vi "new FGGA TCP Packet_v3.3.vi"(0 "ID":string, 5 "Version":string, 7 "TCP Packet In":string, 9 "utc_time":u32, 12 "Data Array":string[](array[string])) -> (8 "TCP Binary Packet":string)   [LabVIEW 2014]
panel:
  out "array":string[](array[string])
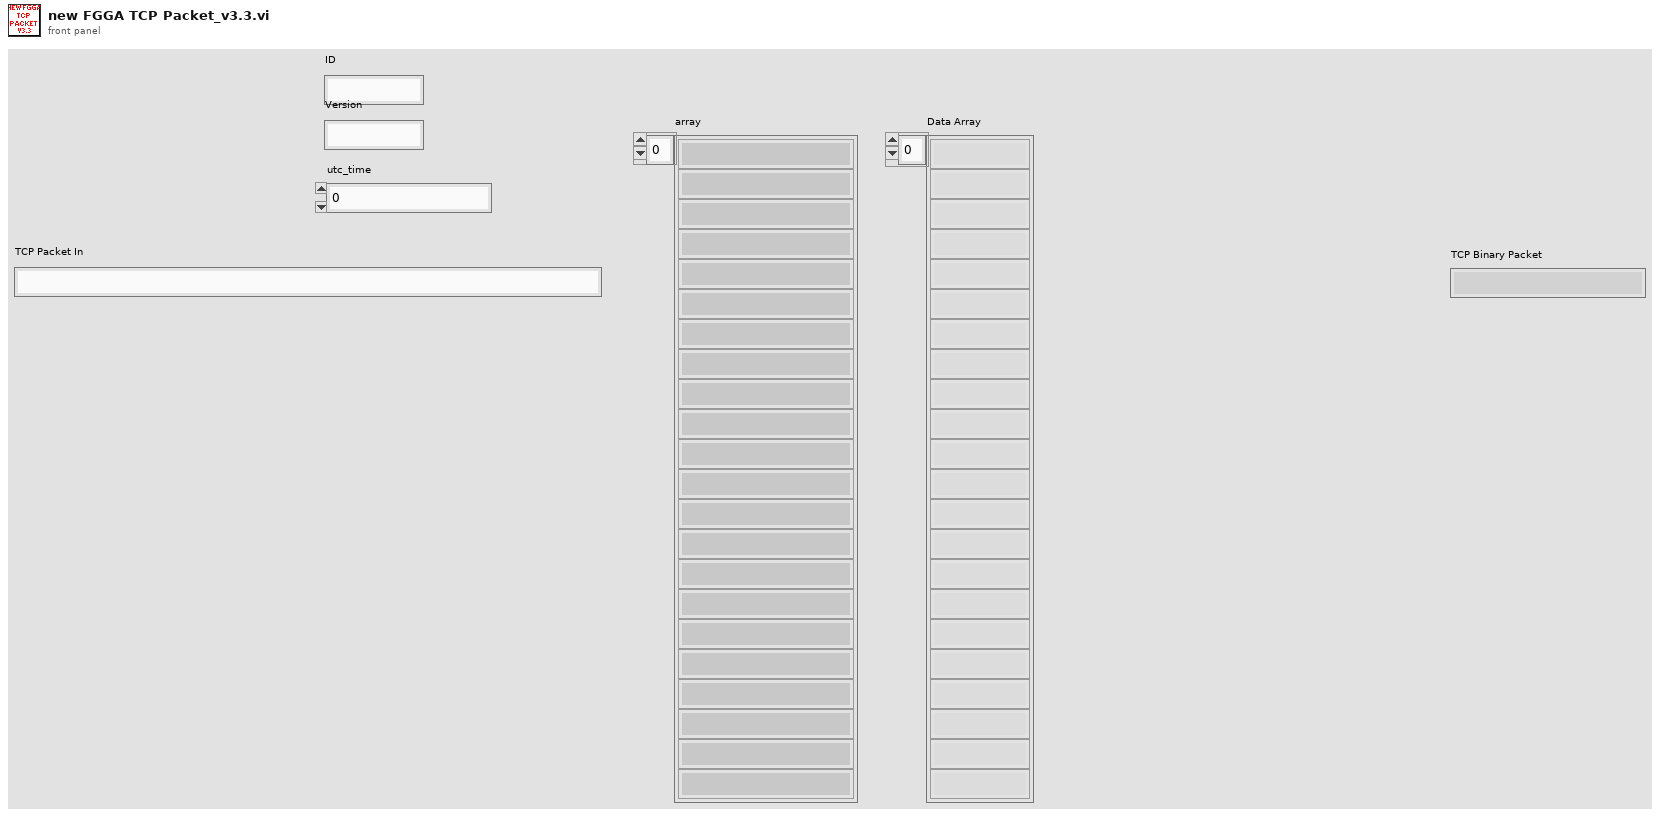
[diagram p1: front panel]
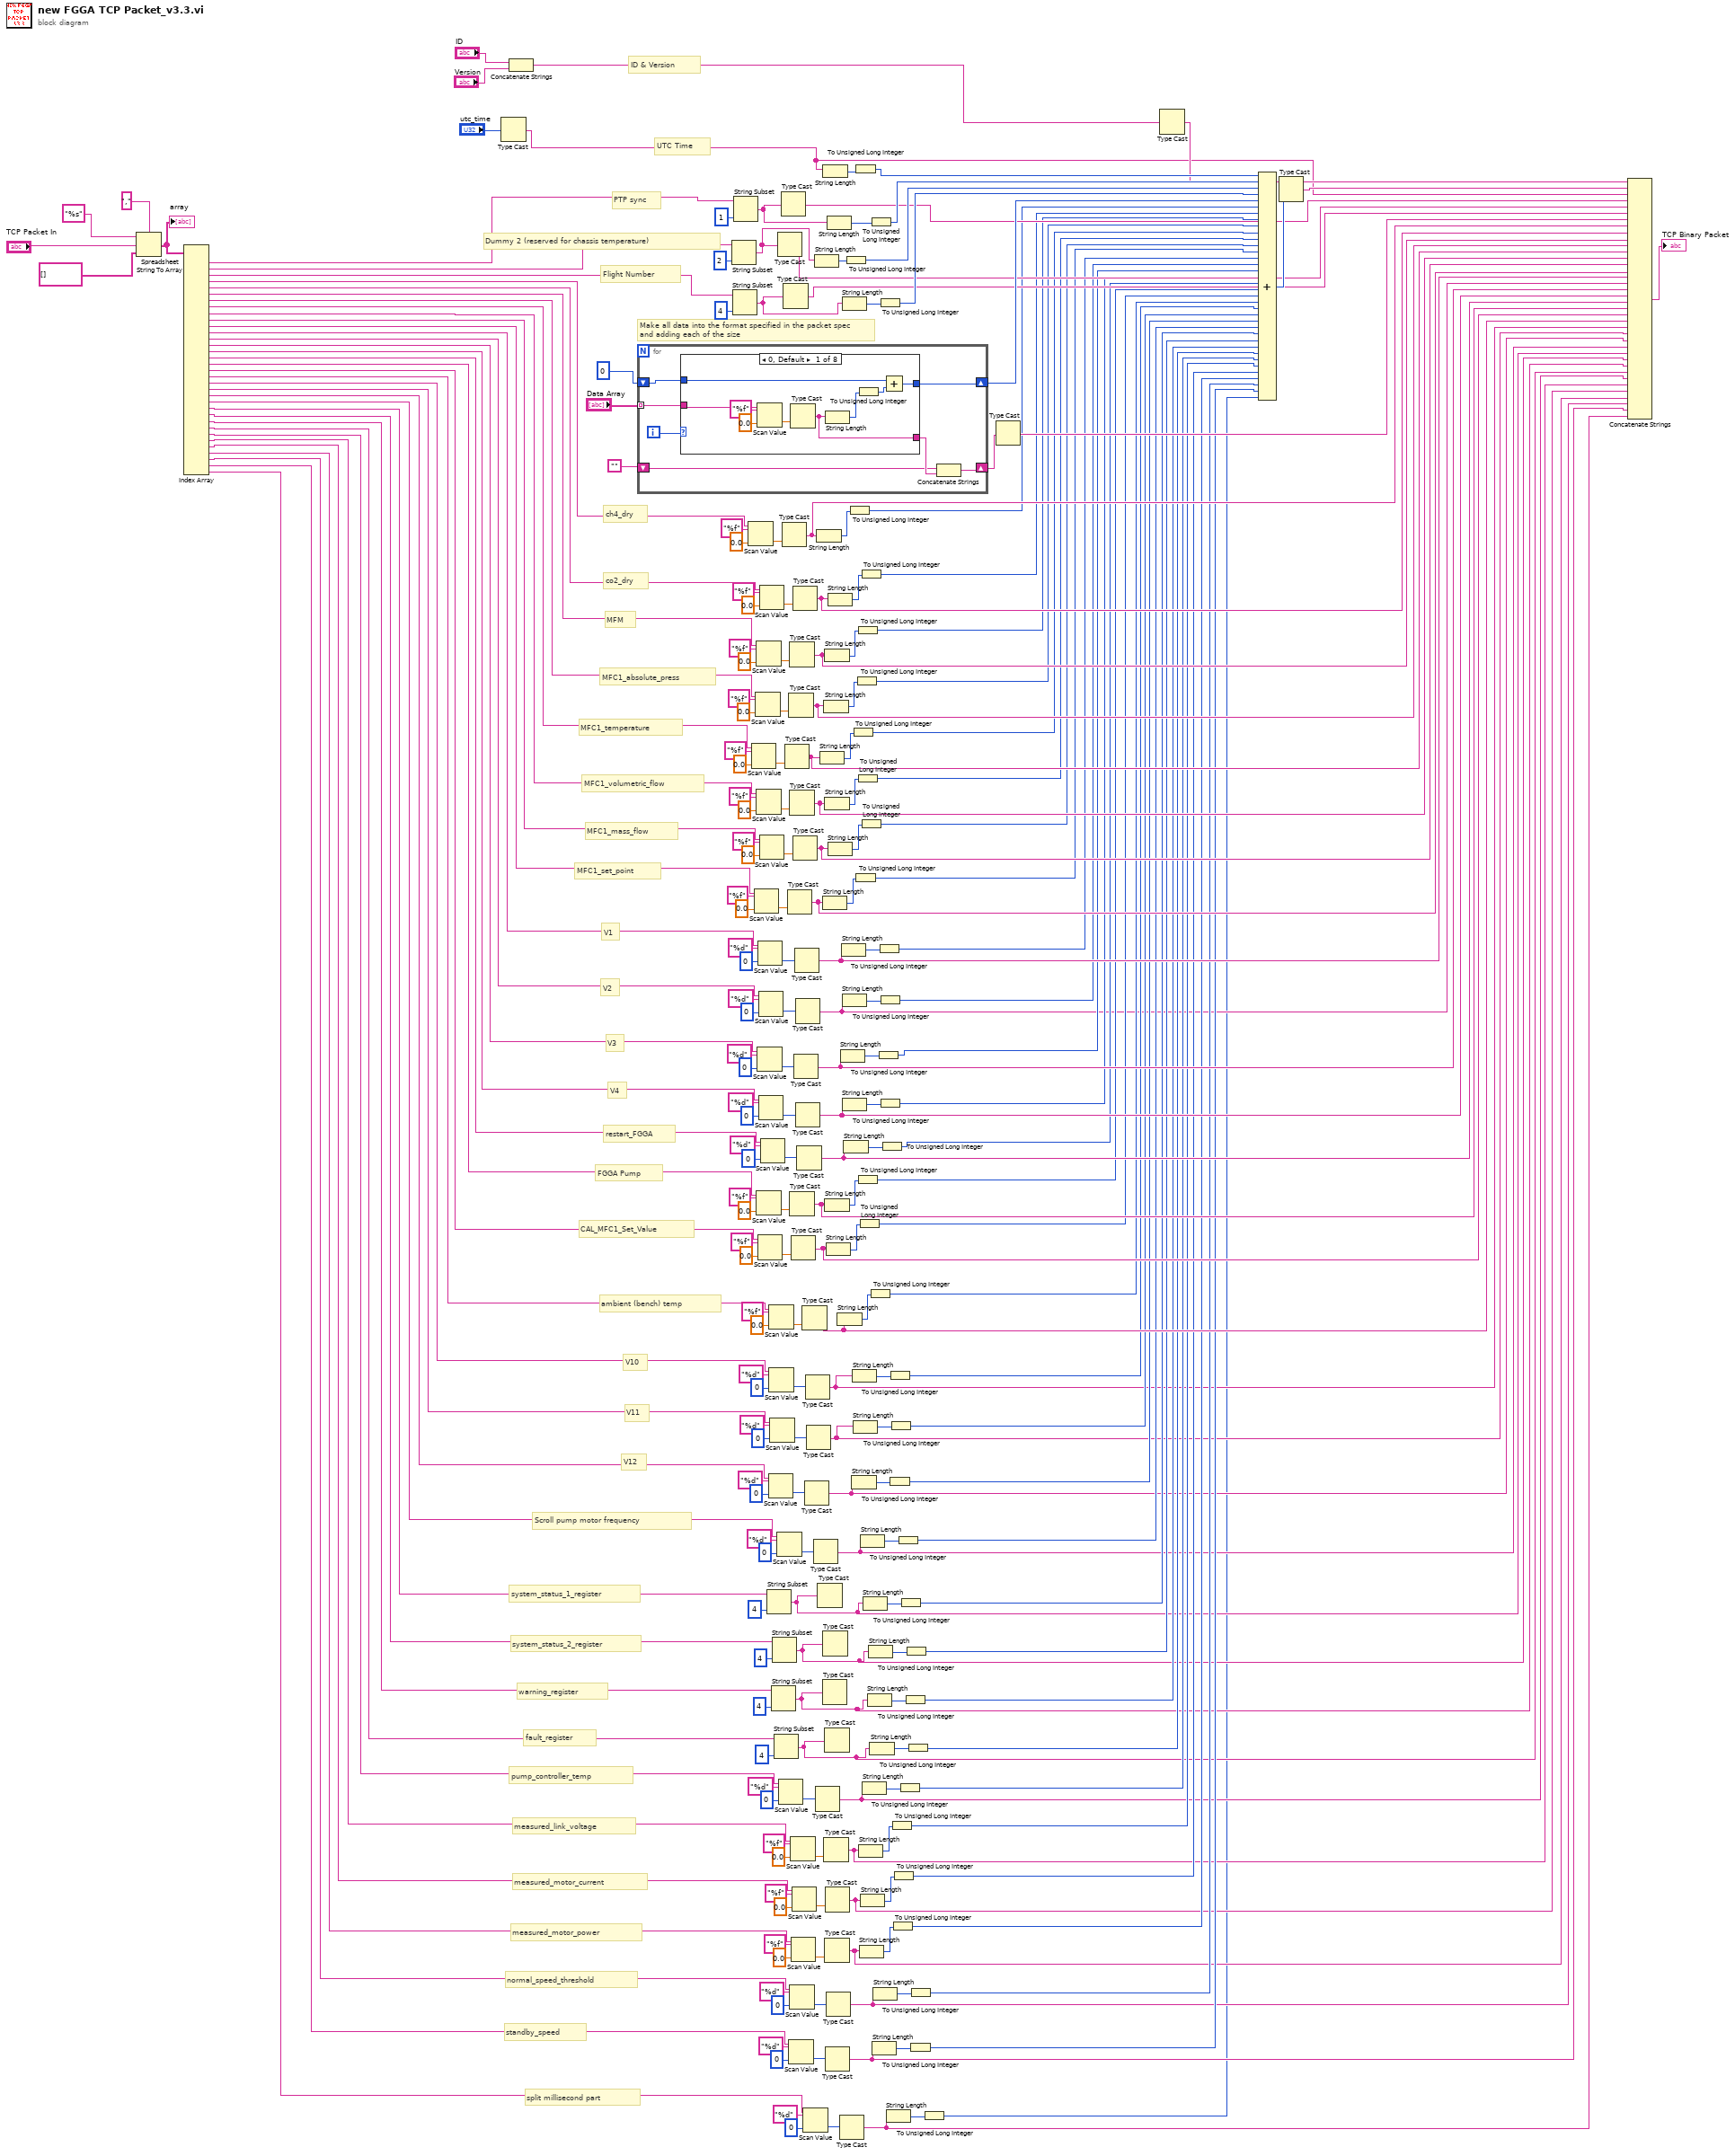
[diagram p0: block diagram]
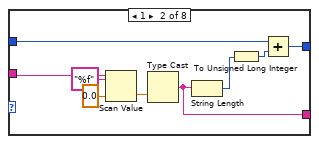
[diagram p2: hidden frame]
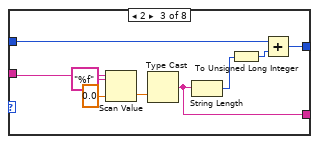
[diagram p3: hidden frame]
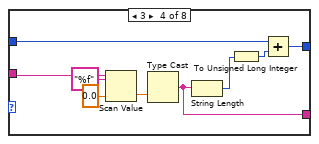
[diagram p4: hidden frame]
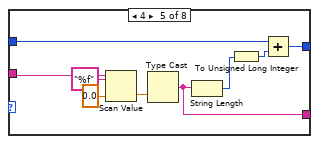
[diagram p5: hidden frame]
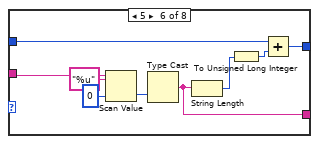
[diagram p6: hidden frame]
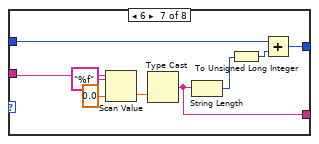
[diagram p7: hidden frame]
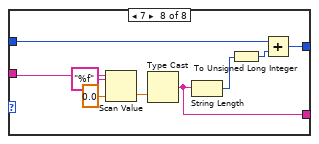
[diagram p8: hidden frame]
diagram:
  # "split millisecond part"
  # "standby_speed"
  # "normal_speed_threshold"
  # "measured_motor_power"
  # "measured_motor_current"
  # "measured_link_voltage"
  # "pump_controller_temp"
  # "fault_register"
  # "warning_register"
  # "system_status_2_register"
  # "system_status_1_register"
  # "Scroll pump motor frequency"
  # "V12"
  # "V11"
  # "V10"
  # "ambient (bench) temp"
  # "PTP sync"
  # "CAL_MFC1_Set_Value"
  # "FGGA Pump"
  # "restart_FGGA"
  # "V4"
  # "V3"
  # "V2"
  # "V1"
  # "MFC1_set_point"
  # "MFC1_mass_flow"
  # "MFC1_volumetric_flow"
  # "MFC1_temperature"
  # "MFC1_absolute_press"
  # "MFM"
  # "co2_dry"
  # "ch4_dry"
  # "Flight Number"
  # "Dummy 2 (reserved for chassis temperature)"
  # "UTC Time"
  # "ID & Version"
  # "Make all data into the format specified in the packet spec\nand adding each of the size"
  n1 = Spreadsheet String To Array(delimiter (Tab)=",", format string="%s", spreadsheet string="TCP Packet In", array type (2D Dbl)=string[] []) -> (array=w206:string[])
  "array" <- w206
  n2 = Index Array(array=w206) -> (element #1=w205:string, element #2=w204:string, element #3=w203:string, element #4=w202:string, element #5=w201:string, element #6=w176:string, element #7=w173:string, element #8=w170:string, element #9=w167:string, element #10=w164:string, element #11=w161:string, element #12=w154:string, element #13=w147:string, element #14=w125:string, element #15=w122:string, element #16=w119:string, element #17=w116:string, element #18=w113:string, element #19=w101:string, element #20=w50:string, element #21=w49:string, element #22=w48:string, element #23=w47:string, element #24=w46:string, element #25=w45:string, element #26=w44:string, element #27=w43:string, element #28=w42:string, element #29=w41:string, element #30=w40:string, element #31=w39:string, element #32=w38:string, element #33=w37:string, element #34=w3:string)  [unwired: 34 in]
  n3 = Type Cast(x="utc_time") -> (*(type *) &x=w106:string)  [unwired: 1 in]
  n4 = Concatenate Strings("ID", "Version") -> (w108:string)
  n5 = for {
    tunnel: "Data Array" -> [w255] mode=indexing
    shift-right: [w253] -> w237
    shift-left: u32 0 -> [w254]
    shift-right: [w252] -> w226
    shift-left: "" -> [w250]
    i -> [w256]
    n6 = case shown="0, Default" w256 {
      tunnel: w255 -> [w263 w272 w281 w290 w299 w308 w317 w326]
      tunnel: w254 -> [w261 w270 w279 w288 w297 w306 w315 w324]
      tunnel: [w258 w267 w276 w285 w294 w303 w312 w321] -> w253
      tunnel: [w257 w266 w275 w284 w293 w302 w311 w320] -> w251
      frame 0, Default {
        n7 = Scan Value(string=w263, format string="%f", default (0 dbl)=sgl 0.0 ("default (0 I32)")) -> (value=w265:sgl)  [unwired: 1 out]
        n8 = Type Cast(x=w265) -> (*(type *) &x=w257:string)  [unwired: 1 in]
        n9 = String Length(string=w257) -> (length=w260:i32)
        n10 = To Unsigned Long Integer(number=w260) -> (unsigned 32bit integer=w259:u32)
        n11 = Add(x=w261, y=w259) -> (x+y=w258:u32)
      }
      frame 1 {
        n12 = Scan Value(string=w272, format string="%f", default (0 dbl)=sgl 0.0 ("default (0 I32)")) -> (value=w274:sgl)  [unwired: 1 out]
        n13 = Type Cast(x=w274) -> (*(type *) &x=w266:string)  [unwired: 1 in]
        n14 = String Length(string=w266) -> (length=w269:i32)
        n15 = To Unsigned Long Integer(number=w269) -> (unsigned 32bit integer=w268:u32)
        n16 = Add(x=w270, y=w268) -> (x+y=w267:u32)
      }
      frame 2 {
        n17 = Scan Value(string=w281, format string="%f", default (0 dbl)=sgl 0.0 ("default (0 I32)")) -> (value=w283:sgl)  [unwired: 1 out]
        n18 = Type Cast(x=w283) -> (*(type *) &x=w275:string)  [unwired: 1 in]
        n19 = String Length(string=w275) -> (length=w278:i32)
        n20 = To Unsigned Long Integer(number=w278) -> (unsigned 32bit integer=w277:u32)
        n21 = Add(x=w279, y=w277) -> (x+y=w276:u32)
      }
      frame 3 {
        n22 = Scan Value(string=w290, format string="%f", default (0 dbl)=sgl 0.0 ("default (0 I32)")) -> (value=w292:sgl)  [unwired: 1 out]
        n23 = Type Cast(x=w292) -> (*(type *) &x=w284:string)  [unwired: 1 in]
        n24 = String Length(string=w284) -> (length=w287:i32)
        n25 = To Unsigned Long Integer(number=w287) -> (unsigned 32bit integer=w286:u32)
        n26 = Add(x=w288, y=w286) -> (x+y=w285:u32)
      }
      frame 4 {
        n27 = Scan Value(string=w299, format string="%f", default (0 dbl)=sgl 0.0 ("default (0 I32)")) -> (value=w301:sgl)  [unwired: 1 out]
        n28 = Type Cast(x=w301) -> (*(type *) &x=w293:string)  [unwired: 1 in]
        n29 = String Length(string=w293) -> (length=w296:i32)
        n30 = To Unsigned Long Integer(number=w296) -> (unsigned 32bit integer=w295:u32)
        n31 = Add(x=w297, y=w295) -> (x+y=w294:u32)
      }
      frame 5 {
        n32 = Scan Value(string=w308, format string="%u", default (0 dbl)=u16 0 ("default (0 I32)")) -> (value=w310:u16)  [unwired: 1 out]
        n33 = Type Cast(x=w310) -> (*(type *) &x=w302:string)  [unwired: 1 in]
        n34 = String Length(string=w302) -> (length=w305:i32)
        n35 = To Unsigned Long Integer(number=w305) -> (unsigned 32bit integer=w304:u32)
        n36 = Add(x=w306, y=w304) -> (x+y=w303:u32)
      }
      frame 6 {
        n37 = Scan Value(string=w317, format string="%f", default (0 dbl)=sgl 0.0 ("default (0 I32)")) -> (value=w319:sgl)  [unwired: 1 out]
        n38 = Type Cast(x=w319) -> (*(type *) &x=w311:string)  [unwired: 1 in]
        n39 = String Length(string=w311) -> (length=w314:i32)
        n40 = To Unsigned Long Integer(number=w314) -> (unsigned 32bit integer=w313:u32)
        n41 = Add(x=w315, y=w313) -> (x+y=w312:u32)
      }
      frame 7 {
        n42 = Scan Value(string=w326, format string="%f", default (0 dbl)=sgl 0.0 ("default (0 I32)")) -> (value=w328:sgl)  [unwired: 1 out]
        n43 = Type Cast(x=w328) -> (*(type *) &x=w320:string)  [unwired: 1 in]
        n44 = String Length(string=w320) -> (length=w323:i32)
        n45 = To Unsigned Long Integer(number=w323) -> (unsigned 32bit integer=w322:u32)
        n46 = Add(x=w324, y=w322) -> (x+y=w321:u32)
      }
    }
    n47 = Concatenate Strings(w250, w251) -> (w252:string)
  }
  n48 = String Subset(string=w204, length (rest)=2 ("length (rest)")) -> (substring=w224:string)  [unwired: 1 in]
  n49 = String Subset(string=w203, length (rest)=4 ("length (rest)")) -> (substring=w230:string)  [unwired: 1 in]
  n50 = String Subset(string=w205, length (rest)=1 ("length (rest)")) -> (substring=w233:string)  [unwired: 1 in]
  n51 = Scan Value(string=w202, format string="%f", default (0 dbl)=sgl 0.0 ("default (0 I32)")) -> (value=w222:sgl)  [unwired: 1 out]
  n52 = Scan Value(string=w170, format string="%f", default (0 dbl)=sgl 0.0 ("default (0 I32)")) -> (value=w192:sgl)  [unwired: 1 out]
  n53 = Scan Value(string=w161, format string="%f", default (0 dbl)=sgl 0.0 ("default (0 I32)")) -> (value=w180:sgl)  [unwired: 1 out]
  n54 = Scan Value(string=w173, format string="%f", default (0 dbl)=sgl 0.0 ("default (0 I32)")) -> (value=w196:sgl)  [unwired: 1 out]
  n55 = Scan Value(string=w176, format string="%f", default (0 dbl)=sgl 0.0 ("default (0 I32)")) -> (value=w200:sgl)  [unwired: 1 out]
  n56 = Scan Value(string=w167, format string="%f", default (0 dbl)=sgl 0.0 ("default (0 I32)")) -> (value=w188:sgl)  [unwired: 1 out]
  n57 = Scan Value(string=w116, format string="%f", default (0 dbl)=sgl 0.0 ("default (0 I32)")) -> (value=w133:sgl)  [unwired: 1 out]
  n58 = Scan Value(string=w125, format string="%d", default (0 dbl)=u16 0 ("default (0 I32)")) -> (value=w142:u16)  [unwired: 1 out]
  n59 = Scan Value(string=w154, format string="%d", default (0 dbl)=u16 0 ("default (0 I32)")) -> (value=w155:u16)  [unwired: 1 out]
  n60 = Scan Value(string=w113, format string="%f", default (0 dbl)=sgl 0.0 ("default (0 I32)")) -> (value=w129:sgl)  [unwired: 1 out]
  n61 = Scan Value(string=w147, format string="%d", default (0 dbl)=u16 0 ("default (0 I32)")) -> (value=w148:u16)  [unwired: 1 out]
  n62 = Scan Value(string=w122, format string="%d", default (0 dbl)=u16 0 ("default (0 I32)")) -> (value=w138:u16)  [unwired: 1 out]
  n63 = Scan Value(string=w201, format string="%f", default (0 dbl)=sgl 0.0 ("default (0 I32)")) -> (value=w216:sgl)  [unwired: 1 out]
  n64 = Scan Value(string=w164, format string="%f", default (0 dbl)=sgl 0.0 ("default (0 I32)")) -> (value=w184:sgl)  [unwired: 1 out]
  n65 = Scan Value(string=w119, format string="%d", default (0 dbl)=u16 0 ("default (0 I32)")) -> (value=w134:u16)  [unwired: 1 out]
  n66 = String Subset(string=w46, length (rest)=4 ("length (rest)")) -> (substring=w18:string)  [unwired: 1 in]
  n67 = Scan Value(string=w48, format string="%d", default (0 dbl)=u16 0 ("default (0 I32)")) -> (value=w87:u16)  [unwired: 1 out]
  n68 = Scan Value(string=w101, format string="%f", default (0 dbl)=sgl 0.0 ("default (0 I32)")) -> (value=w105:sgl)  [unwired: 1 out]
  n69 = Scan Value(string=w50, format string="%d", default (0 dbl)=u16 0 ("default (0 I32)")) -> (value=w95:u16)  [unwired: 1 out]
  n70 = Scan Value(string=w49, format string="%d", default (0 dbl)=u16 0 ("default (0 I32)")) -> (value=w91:u16)  [unwired: 1 out]
  n71 = String Subset(string=w44, length (rest)=4 ("length (rest)")) -> (substring=w17:string)  [unwired: 1 in]
  n72 = String Subset(string=w45, length (rest)=4 ("length (rest)")) -> (substring=w5:string)  [unwired: 1 in]
  n73 = String Subset(string=w43, length (rest)=4 ("length (rest)")) -> (substring=w16:string)  [unwired: 1 in]
  n74 = Scan Value(string=w47, format string="%d", default (0 dbl)=u16 0 ("default (0 I32)")) -> (value=w83:u16)  [unwired: 1 out]
  n75 = Type Cast(x=w224) -> (*(type *) &x=w223:string)  [unwired: 1 in]
  n76 = Scan Value(string=w42, format string="%d", default (0 dbl)=u16 0 ("default (0 I32)")) -> (value=w71:u16)  [unwired: 1 out]
  n77 = Type Cast(x=w233) -> (*(type *) &x=w232:string)  [unwired: 1 in]
  n78 = Type Cast(x=w222) -> (*(type *) &x=w218:string)  [unwired: 1 in]
  n79 = Type Cast(x=w230) -> (*(type *) &x=w231:string)  [unwired: 1 in]
  n80 = Type Cast(x=w192) -> (*(type *) &x=w168:string)  [unwired: 1 in]
  n81 = Type Cast(x=w180) -> (*(type *) &x=w159:string)  [unwired: 1 in]
  n82 = Type Cast(x=w196) -> (*(type *) &x=w171:string)  [unwired: 1 in]
  n83 = Scan Value(string=w37, format string="%d", default (0 dbl)=u16 0 ("default (0 I32)")) -> (value=w51:u16)  [unwired: 1 out]
  n84 = Type Cast(x=w200) -> (*(type *) &x=w174:string)  [unwired: 1 in]
  n85 = Type Cast(x=w188) -> (*(type *) &x=w165:string)  [unwired: 1 in]
  n86 = Type Cast(x=w133) -> (*(type *) &x=w114:string)  [unwired: 1 in]
  n87 = Scan Value(string=w38, format string="%d", default (0 dbl)=u16 0 ("default (0 I32)")) -> (value=w55:u16)  [unwired: 1 out]
  n88 = Scan Value(string=w41, format string="%f", default (0 dbl)=sgl 0.0 ("default (0 I32)")) -> (value=w70:sgl)  [unwired: 1 out]
  n89 = Type Cast(x=w129) -> (*(type *) &x=w111:string)  [unwired: 1 in]
  n90 = Scan Value(string=w39, format string="%f", default (0 dbl)=sgl 0.0 ("default (0 I32)")) -> (value=w62:sgl)  [unwired: 1 out]
  n91 = Scan Value(string=w40, format string="%f", default (0 dbl)=sgl 0.0 ("default (0 I32)")) -> (value=w66:sgl)  [unwired: 1 out]
  n92 = Type Cast(x=w216) -> (*(type *) &x=w211:string)  [unwired: 1 in]
  n93 = Type Cast(x=w184) -> (*(type *) &x=w162:string)  [unwired: 1 in]
  n94 = Type Cast(x=w142) -> (*(type *) &x=w123:string)  [unwired: 1 in]
  n95 = Type Cast(x=w155) -> (*(type *) &x=w152:string)  [unwired: 1 in]
  n96 = Type Cast(x=w148) -> (*(type *) &x=w4:string)  [unwired: 1 in]
  n97 = Type Cast(x=w138) -> (*(type *) &x=w120:string)  [unwired: 1 in]
  n98 = Type Cast(x=w134) -> (*(type *) &x=w117:string)  [unwired: 1 in]
  n99 = Type Cast(x=w105) -> (*(type *) &x=w99:string)  [unwired: 1 in]
  n100 = Scan Value(string=w3, format string="%d", default (0 dbl)=u16 0 ("default (0 I32)")) -> (value=w6:u16)  [unwired: 1 out]
  n101 = Type Cast(x=w87) -> (*(type *) &x=w20:string)  [unwired: 1 in]
  n102 = Type Cast(x=w95) -> (*(type *) &x=w22:string)  [unwired: 1 in]
  n103 = Type Cast(x=w91) -> (*(type *) &x=w21:string)  [unwired: 1 in]
  n104 = Type Cast(x=w83) -> (*(type *) &x=w19:string)  [unwired: 1 in]
  n105 = String Length(string=w224) -> (length=w244:i32)
  n106 = Type Cast(x=w71) -> (*(type *) &x=w15:string)  [unwired: 1 in]
  n107 = String Length(string=w218) -> (length=w219:i32)
  n108 = Type Cast(x=w18) -> ()  [unwired: 1 in, 1 out]
  n109 = String Length(string=w168) -> (length=w189:i32)
  n110 = String Length(string=w159) -> (length=w177:i32)
  n111 = Type Cast(x=w17) -> ()  [unwired: 1 in, 1 out]
  n112 = String Length(string=w106) -> (length=w249:i32)
  n113 = Type Cast(x=w5) -> ()  [unwired: 1 in, 1 out]
  n114 = String Length(string=w171) -> (length=w193:i32)
  n115 = Type Cast(x=w70) -> (*(type *) &x=w14:string)  [unwired: 1 in]
  n116 = String Length(string=w174) -> (length=w197:i32)
  n117 = String Length(string=w165) -> (length=w185:i32)
  n118 = String Length(string=w114) -> (length=w130:i32)
  n119 = Type Cast(x=w16) -> ()  [unwired: 1 in, 1 out]
  n120 = Type Cast(x=w62) -> (*(type *) &x=w13:string)  [unwired: 1 in]
  n121 = Type Cast(x=w66) -> (*(type *) &x=w11:string)  [unwired: 1 in]
  n122 = Type Cast(x=w51) -> (*(type *) &x=w10:string)  [unwired: 1 in]
  n123 = String Length(string=w111) -> (length=w126:i32)
  n124 = Type Cast(x=w55) -> (*(type *) &x=w12:string)  [unwired: 1 in]
  n125 = String Length(string=w233) -> (length=w246:i32)
  n126 = String Length(string=w211) -> (length=w213:i32)
  n127 = String Length(string=w162) -> (length=w181:i32)
  n128 = String Length(string=w99) -> (length=w102:i32)
  n129 = Type Cast(x=w6) -> (*(type *) &x=w1:string)  [unwired: 1 in]
  n130 = String Length(string=w123) -> (length=w145:i32)
  n131 = String Length(string=w152) -> (length=w158:i32)
  n132 = String Length(string=w230) -> (length=w241:i32)
  n133 = String Length(string=w4) -> (length=w151:i32)
  n134 = String Length(string=w120) -> (length=w141:i32)
  n135 = To Unsigned Long Integer(number=w244) -> (unsigned 32bit integer=w243:u32)
  n136 = String Length(string=w117) -> (length=w137:i32)
  n137 = To Unsigned Long Integer(number=w219) -> (unsigned 32bit integer=w217:u32)
  n138 = To Unsigned Long Integer(number=w189) -> (unsigned 32bit integer=w169:u32)
  n139 = String Length(string=w20) -> (length=w90:i32)
  n140 = String Length(string=w22) -> (length=w98:i32)
  n141 = To Unsigned Long Integer(number=w249) -> (unsigned 32bit integer=w248:u32)
  n142 = To Unsigned Long Integer(number=w177) -> (unsigned 32bit integer=w160:u32)
  n143 = String Length(string=w21) -> (length=w94:i32)
  n144 = To Unsigned Long Integer(number=w193) -> (unsigned 32bit integer=w172:u32)
  n145 = To Unsigned Long Integer(number=w197) -> (unsigned 32bit integer=w175:u32)
  n146 = To Unsigned Long Integer(number=w185) -> (unsigned 32bit integer=w166:u32)
  n147 = To Unsigned Long Integer(number=w130) -> (unsigned 32bit integer=w115:u32)
  n148 = To Unsigned Long Integer(number=w126) -> (unsigned 32bit integer=w112:u32)
  n149 = To Unsigned Long Integer(number=w213) -> (unsigned 32bit integer=w212:u32)
  n150 = To Unsigned Long Integer(number=w181) -> (unsigned 32bit integer=w163:u32)
  n151 = String Length(string=w14) -> (length=w67:i32)
  n152 = String Length(string=w13) -> (length=w59:i32)
  n153 = String Length(string=w19) -> (length=w86:i32)
  n154 = String Length(string=w11) -> (length=w63:i32)
  n155 = String Length(string=w15) -> (length=w74:i32)
  n156 = String Length(string=w18) -> (length=w81:i32)
  n157 = String Length(string=w17) -> (length=w77:i32)
  n158 = To Unsigned Long Integer(number=w102) -> (unsigned 32bit integer=w100:u32)
  n159 = String Length(string=w5) -> (length=w79:i32)
  n160 = To Unsigned Long Integer(number=w246) -> (unsigned 32bit integer=w245:u32)
  n161 = String Length(string=w16) -> (length=w75:i32)
  n162 = String Length(string=w10) -> (length=w54:i32)
  n163 = String Length(string=w12) -> (length=w58:i32)
  n164 = To Unsigned Long Integer(number=w145) -> (unsigned 32bit integer=w124:u32)
  n165 = To Unsigned Long Integer(number=w158) -> (unsigned 32bit integer=w153:u32)
  n166 = To Unsigned Long Integer(number=w241) -> (unsigned 32bit integer=w240:u32)
  n167 = To Unsigned Long Integer(number=w151) -> (unsigned 32bit integer=w146:u32)
  n168 = To Unsigned Long Integer(number=w141) -> (unsigned 32bit integer=w121:u32)
  n169 = To Unsigned Long Integer(number=w137) -> (unsigned 32bit integer=w118:u32)
  n170 = String Length(string=w1) -> (length=w9:i32)
  n171 = To Unsigned Long Integer(number=w90) -> (unsigned 32bit integer=w34:u32)
  n172 = To Unsigned Long Integer(number=w98) -> (unsigned 32bit integer=w36:u32)
  n173 = To Unsigned Long Integer(number=w94) -> (unsigned 32bit integer=w35:u32)
  n174 = To Unsigned Long Integer(number=w67) -> (unsigned 32bit integer=w27:u32)
  n175 = To Unsigned Long Integer(number=w59) -> (unsigned 32bit integer=w25:u32)
  n176 = To Unsigned Long Integer(number=w63) -> (unsigned 32bit integer=w26:u32)
  n177 = To Unsigned Long Integer(number=w86) -> (unsigned 32bit integer=w33:u32)
  n178 = To Unsigned Long Integer(number=w74) -> (unsigned 32bit integer=w28:u32)
  n179 = To Unsigned Long Integer(number=w81) -> (unsigned 32bit integer=w32:u32)
  n180 = To Unsigned Long Integer(number=w77) -> (unsigned 32bit integer=w30:u32)
  n181 = To Unsigned Long Integer(number=w79) -> (unsigned 32bit integer=w31:u32)
  n182 = To Unsigned Long Integer(number=w75) -> (unsigned 32bit integer=w29:u32)
  n183 = To Unsigned Long Integer(number=w54) -> (unsigned 32bit integer=w23:u32)
  n184 = To Unsigned Long Integer(number=w58) -> (unsigned 32bit integer=w24:u32)
  n185 = To Unsigned Long Integer(number=w9) -> (unsigned 32bit integer=w2:u32)
  n186 = Type Cast(x=w226) -> (*(type *) &x=w229:string)  [unwired: 1 in]
  n187 = Type Cast(x=w108) -> (*(type *) &x=w236:string)  [unwired: 1 in]
  n188 = Compound Arithmetic op=ADD(w248, w245, w243, w240, w237, w217, w212, w175, w172, w169, w166, w163, w160, w153, w146, w124, w121, w118, w115, w112, w100, w36, w35, w34, w33, w32, w31, w30, w29, w28, w27, w26, w25, w24, w23, w2) -> (w235:u32)
  n189 = Type Cast(x=w235) -> (*(type *) &x=w234:string)  [unwired: 1 in]
  n190 = Concatenate Strings(w236, w234, w106, w232, w223, w231, w229, w218, w211, w174, w171, w168, w165, w162, w159, w152, w4, w123, w120, w117, w114, w111, w99, w22, w21, w20, w19, w18, w5, w17, w16, w15, w14, w11, w13, w12, w10, w1) -> (→"TCP Binary Packet":string)
